vi "Transcript VIs and Upload.vi"() -> ()   [LabVIEW 2014]
uses:
  <vilib>/LabVIEW Universal Transcriptor/LabVIEW to Arduino Transcriptor/types/LabVIEW Universal Transcriptor Arduino Boards Specific Names.ctl
panel:
  out "standard output":string
  out "standard error":string
  out "transcripted code":string
  out "error out":errorcluster
  in  "VISA resource name":refnum<visa-resource-name>="COM3"
  in  "vi path":path
  in  "Arduino IDE installation directory":path=path "c:/Program Files/Arduino/arduino.exe "
  in  "Board type":T1="arduino:avr:nano"
  in  "error in":errorcluster
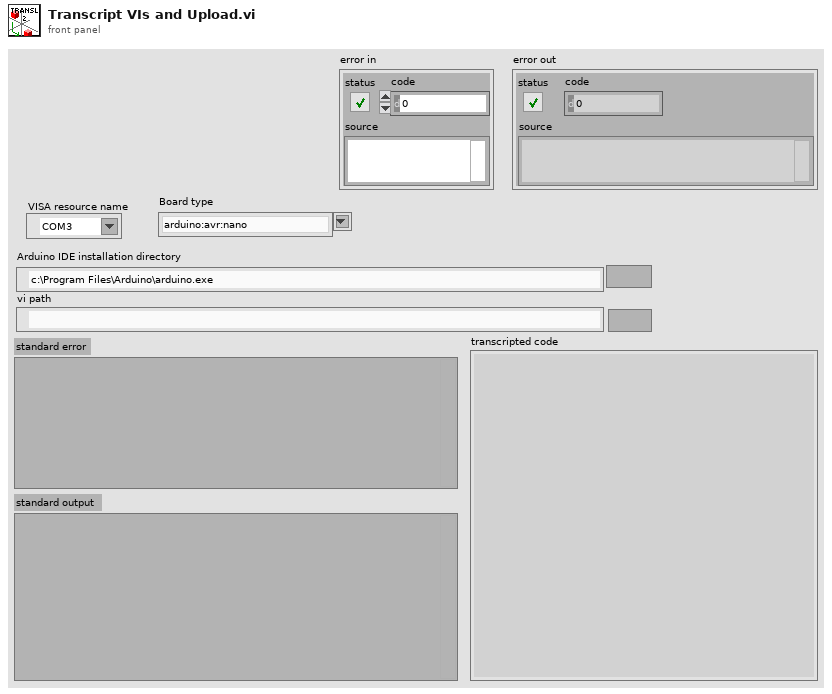
[diagram p1: front panel]
types:
  T1 = typedef "LabVIEW Universal Transcriptor Arduino Boards Specific Names.ctl" = string
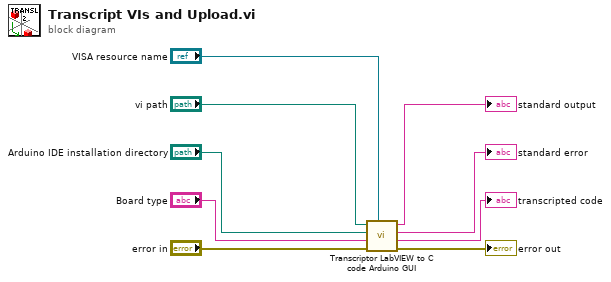
[diagram p0: block diagram]
diagram:
  n1 = call <vilib>:"Transcriptor LabVIEW to C code Arduino GUI.vi"("VISA resource name"="VISA resource name", "error in (no error)"="error in", "Board type"="Board type", "Arduino IDE installation directory"="Arduino IDE installation directory", "vi path"="vi path") -> ("error out"=→"error out":errorcluster, "transcripted code"=→"transcripted code":string, "standard error"=→"standard error":string, "standard output"=→"standard output":string)  [unwired: 3 in]
